vi "Fail QTY VI.vi"(9 "ok":path, 11 "file path (use dialog)":path) -> (3 "path":path)   [LabVIEW 2013]
panel:
  out "path 2":path
  out "array":string[](array[string])
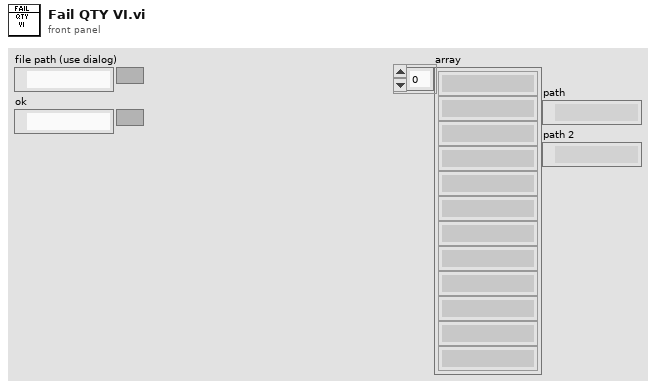
[diagram p1: front panel]
types:
  T1 = enum16{"open", "replace", "create", "open or create", "replace or create", "replace or create with confirmation"}
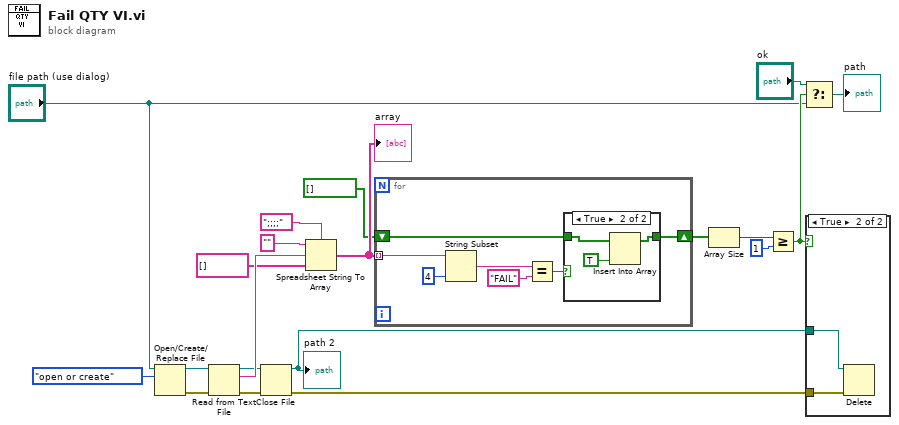
[diagram p0: block diagram]
diagram:
  n1 = Open/Create/Replace File(file path (use dialog)="file path (use dialog)", operation (0:open)=T1."open or create") -> (refnum out=w20:refnum<file>, error out=w10:errorcluster)  [unwired: 4 in, 1 out]
  n2 = Read from Text File(file (use dialog)=w20, error in=w10) -> (refnum out=w4:refnum<file>, text=w19:string, error out=w3:errorcluster)  [unwired: 2 in, 1 out]
  n3 = Close File(refnum=w4, error in=w3) -> (path=w2:path, error out=w1:errorcluster)
  "path 2" <- w2
  n4 = Spreadsheet String To Array(delimiter (Tab)=";;;;", format string="", spreadsheet string=w19, array type (2D Dbl)=string[] []) -> (array=w15:string[])
  "array" <- w15
  n5 = for {
    tunnel: w15 -> [w23] mode=indexing
    shift-right: [w24] -> w13
    shift-left: bool[] [] -> [w26]
    n6 = String Subset(string=w23, length (rest)=4 ("length (rest)")) -> (substring=w22:string)  [unwired: 1 in]
    n7 = Equal?(x=w22, y="FAIL") -> (x = y?=w25:bool)
    n8 = case shown="True" w25 {
      tunnel: w26 -> [w28 w31]
      tunnel: [w28 w29] -> w24
      frame False {
      }
      frame True {
        n9 = Insert Into Array(array=w31, new element=TRUE ("new element/subarray")) -> (w29:bool[])  [unwired: 1 in]
      }
    }
  }
  n10 = Array Size(array=w13) -> (size(s)=w12:i32)
  n11 = Greater Or Equal?(x=w12, y=1) -> (x >= y?=w6:bool)
  n12 = Select(t="ok", s=w6, f="file path (use dialog)") -> (s? t:f=→"path":path)
  n13 = case shown="True" w6 {
    tunnel: w2 -> [_ w33]
    tunnel: w1 -> [_ w32]
    frame False {
    }
    frame True {
      n14 = Delete(path (use dialog)=w33, error in=w32) -> ()  [unwired: 3 in, 3 out]
    }
  }
